vi "UnBundleAndCluster.vi"() -> ()   [LabVIEW 2020]
panel:
  in  "Cluster":cluster{"Name":string, "Age":dbl}
  out "Age":dbl
  out "Name":string
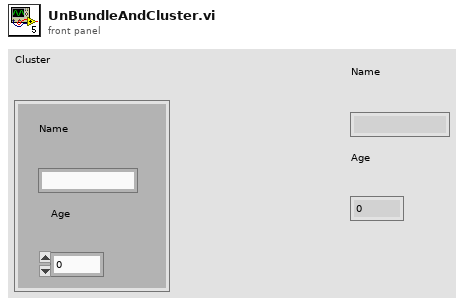
[diagram p1: front panel]
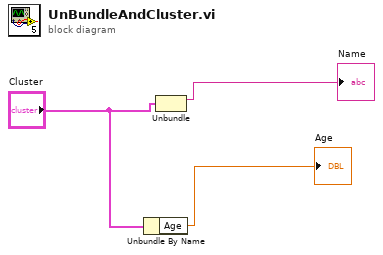
[diagram p0: block diagram]
diagram:
  n1 = Unbundle By Name("Cluster") -> ("Age"=→"Age":dbl)
  n2 = Unbundle("Cluster") -> ("Name"=→"Name":string)  [unwired: 1 out]
